vi "LockinRead.vi"() -> ()   [LabVIEW 2019]
uses:
  SineGlobals.vi
panel:
  out "SENS?":dbl
  out "Freq":dbl
  out "Time Const":dbl
  in  "Query":bool
  out "R [Ohm]":dbl
  in  "Auto Gain":bool
  in  "Auto Phase":bool
  in  "Abort":bool
  in  "Arm":bool
  in  "Peak Amp":dbl=1e-05 format="%#_6e"
  in  "Freq":dbl=71.34 format="%#_6e"
  in  "Numeric":i32=300
  out "Waveform Chart":dbl(graph)
  in  "Lockin Name":refnum<visa-resource-name>="GPIB1::8::INSTR"
  in  "Measure":bool
  out "read buffer":string
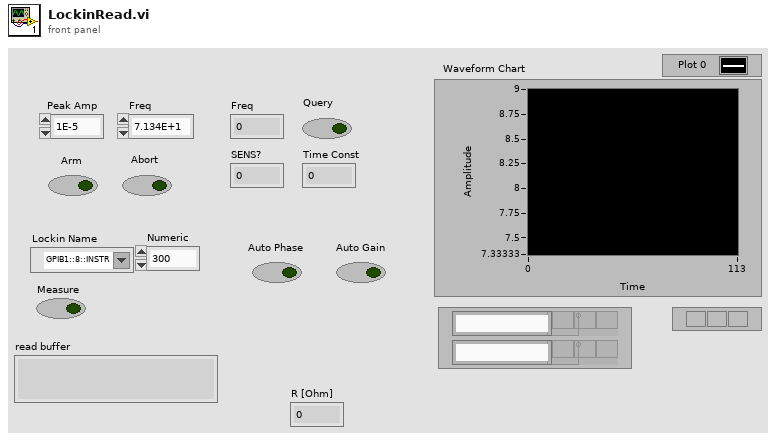
[diagram p1: front panel]
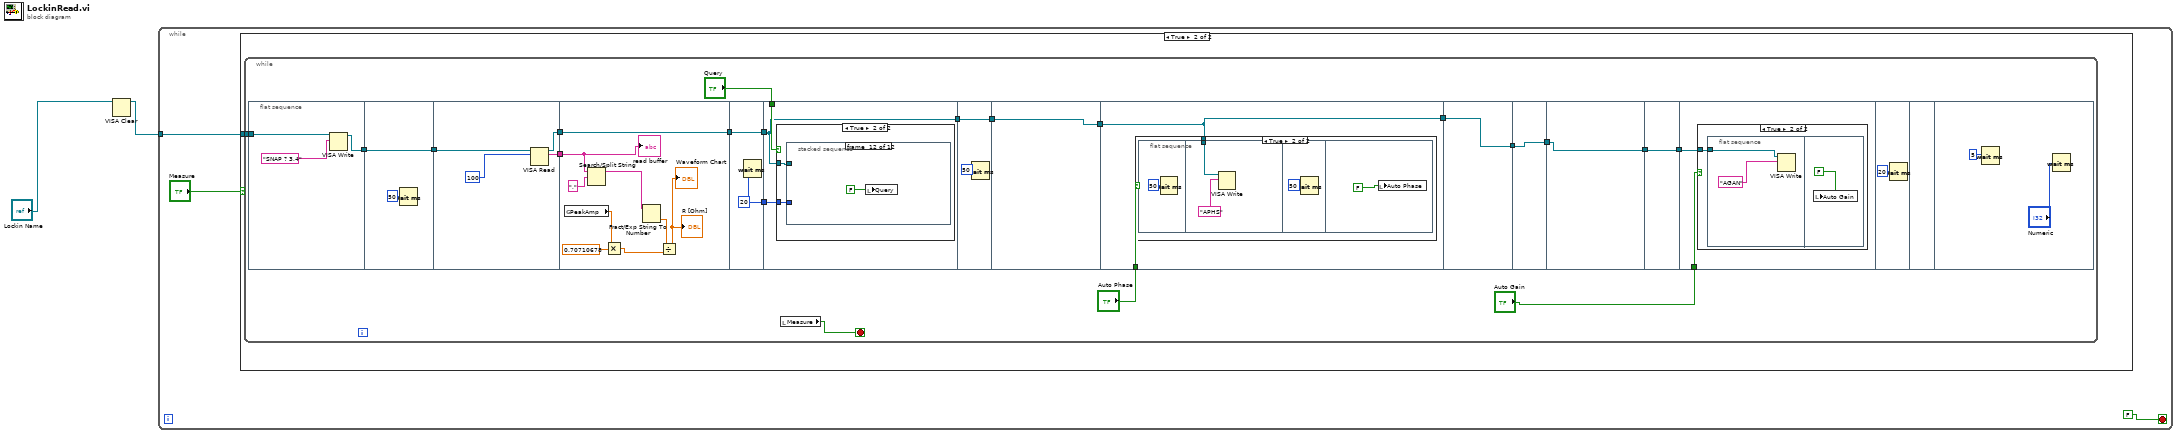
[diagram p0: block diagram]
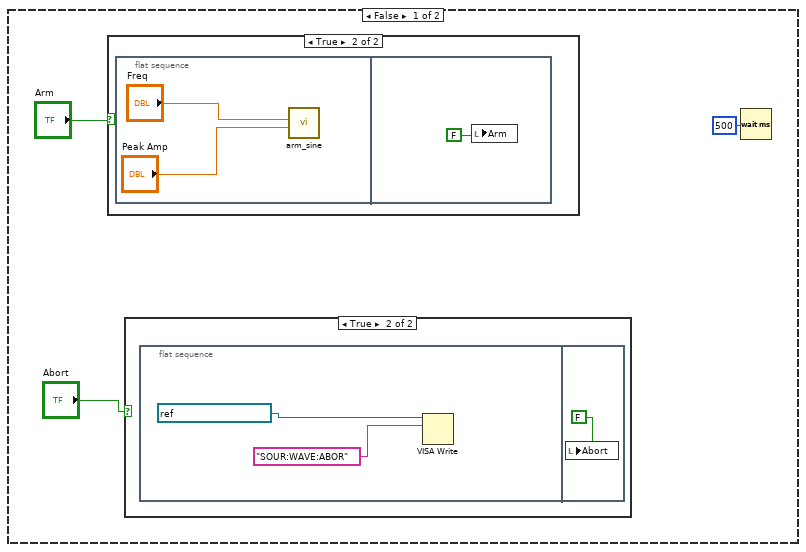
[diagram p2: hidden frame]
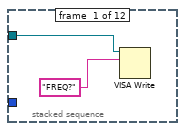
[diagram p6: hidden frame]
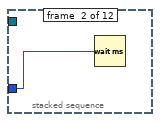
[diagram p7: hidden frame]
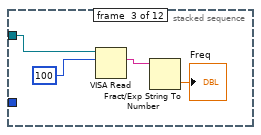
[diagram p8: hidden frame]
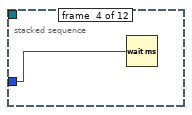
[diagram p9: hidden frame]
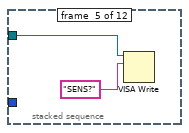
[diagram p10: hidden frame]
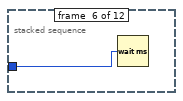
[diagram p11: hidden frame]
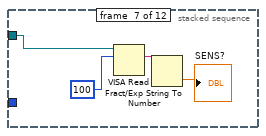
[diagram p12: hidden frame]
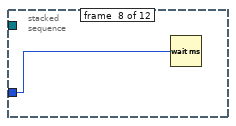
[diagram p13: hidden frame]
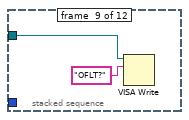
[diagram p14: hidden frame]
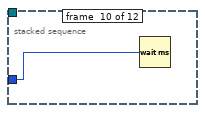
[diagram p15: hidden frame]
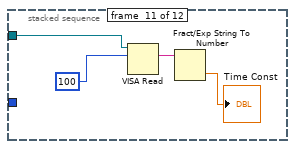
[diagram p16: hidden frame]
diagram:
  n1 = VISA Clear(VISA resource name="Lockin Name") -> (VISA resource name out=w2:refnum<visa-resource-name>)  [unwired: 1 in, 1 out]
  n2 = while {
    tunnel: w2 -> [w3]
    stop <- FALSE stop-if-true
    n3 = case shown="True" "Measure" {
      tunnel: w3 -> [_ w15]
      frame False {
        n4 = case shown="True" "Arm" {
          frame False {
          }
          frame True {
            n5 = flat-sequence {
              frame #0 {
                n6 = call "arm_sine.vi"("Peak Amp"="Peak Amp", "Freq"="Freq") -> ()  [unwired: 10 in]
              }
              frame #1 {
                n7 = local write "Arm"(FALSE) -> ()
              }
            }
          }
        }
        n8 = case shown="True" "Abort" {
          frame False {
          }
          frame True {
            n9 = flat-sequence {
              frame #0 {
                n10 = VISA Write(VISA resource name=refnum<visa-resource-name> "GPIB1::20::INSTR" ("Keithley"), write buffer="SOUR:WAVE:ABOR") -> ()  [unwired: 1 in, 3 out]
              }
              frame #1 {
                n11 = local write "Abort"(FALSE) -> ()
              }
            }
          }
        }
        n12 = Wait (ms)(milliseconds to wait=500) -> ()  [unwired: 1 out]
      }
      frame True {
        n13 = while {
          tunnel: w15 -> [w35]
          stop <- w31 stop-if-true
          n14 = flat-sequence {
            tunnel: w35 -> [w37]
            tunnel: [w36] -> w33
            tunnel: [w40] -> w34
            tunnel: w33 -> [w40]
            tunnel: w34 -> [w44]
            tunnel: [w42] -> w32
            tunnel: [w41] -> w30
            tunnel: w32 -> [w53]
            tunnel: w30 -> [w45]
            tunnel: [w45] -> w29
            tunnel: w29 -> [w55]
            tunnel: [w55] -> w28
            tunnel: [w54] -> w19
            tunnel: w28 -> [w56]
            tunnel: "Query" -> [w58]
            tunnel: w19 -> [w57]
            tunnel: [w56] -> w17
            tunnel: [w85] -> w18
            tunnel: w17 -> [w85]
            tunnel: [w87] -> w27
            tunnel: w18 -> [w87]
            tunnel: w27 -> [w88]
            tunnel: "Auto Phase" -> [w89]
            tunnel: [w88] -> w25
            tunnel: w25 -> [w96]
            tunnel: [w96] -> w16
            tunnel: [w97] -> w24
            tunnel: w16 -> [w97]
            tunnel: w24 -> [w98]
            tunnel: [w98] -> w23
            tunnel: w23 -> [w99]
            tunnel: [w99] -> w22
            tunnel: "Auto Gain" -> [w101]
            tunnel: w22 -> [w100]
            frame #0 {
              n15 = VISA Write(VISA resource name=w37, write buffer="SNAP ? 3,4") -> (VISA resource name out=w36:refnum<visa-resource-name>)  [unwired: 1 in, 2 out]
            }
            frame #1 {
              n16 = Wait (ms)(milliseconds to wait=50) -> ()  [unwired: 1 out]
            }
            frame #2 {
              n17 = VISA Read(VISA resource name=w44, byte count=100) -> (VISA resource name out=w41:refnum<visa-resource-name>, read buffer=w42:string)  [unwired: 1 in, 2 out]
            }
            frame #3 {
              n18 = global read "SineGlobals.vi" "PeakAmp"() -> (w49:dbl)
              n19 = Search/Split String(string=w53, search string/char (-)=",") -> (substring before match=w51:string)  [unwired: 1 in, 2 out]
              n20 = Multiply(x=w49, y=0.70710678) -> (x*y=w46:dbl)
              n21 = Fract/Exp String To Number(string=w51) -> (number=w48:dbl)  [unwired: 3 in, 1 out]
              n22 = Divide(x=w48, y=w46) -> (x/y=→"Waveform Chart" →"R [Ohm]":dbl)
              "read buffer" <- w53
            }
            frame #4 {
              w54 = 20
              n23 = Wait (ms)(milliseconds to wait=w54) -> ()  [unwired: 1 out]
            }
            frame #5 {
              n24 = case shown="True" w58 {
                tunnel: w56 -> [_ w60]
                tunnel: w57 -> [_ w59]
                frame False {
                }
                frame True {
                  n25 = stacked-sequence {
                    tunnel: w60 -> [w61 _ w67 _ w69 _ w75 _ w77 _ w82 _]
                    tunnel: w59 -> [_ w63 _ w68 _ w71 _ w76 _ w79 _ _]
                    frame #0 {
                      n26 = VISA Write(VISA resource name=w61, write buffer="FREQ?") -> ()  [unwired: 1 in, 3 out]
                    }
                    frame #1 {
                      n27 = Wait (ms)(milliseconds to wait=w63) -> ()  [unwired: 1 out]
                    }
                    frame #2 {
                      n28 = VISA Read(VISA resource name=w67, byte count=100) -> (read buffer=w65:string)  [unwired: 1 in, 3 out]
                      n29 = Fract/Exp String To Number(string=w65) -> (number=→"Freq":dbl)  [unwired: 3 in, 1 out]
                    }
                    frame #3 {
                      n30 = Wait (ms)(milliseconds to wait=w68) -> ()  [unwired: 1 out]
                    }
                    frame #4 {
                      n31 = VISA Write(VISA resource name=w69, write buffer="SENS?") -> ()  [unwired: 1 in, 3 out]
                    }
                    frame #5 {
                      n32 = Wait (ms)(milliseconds to wait=w71) -> ()  [unwired: 1 out]
                    }
                    frame #6 {
                      n33 = VISA Read(VISA resource name=w75, byte count=100) -> (read buffer=w73:string)  [unwired: 1 in, 3 out]
                      n34 = Fract/Exp String To Number(string=w73) -> (number=→"SENS?":dbl)  [unwired: 3 in, 1 out]
                    }
                    frame #7 {
                      n35 = Wait (ms)(milliseconds to wait=w76) -> ()  [unwired: 1 out]
                    }
                    frame #8 {
                      n36 = VISA Write(VISA resource name=w77, write buffer="OFLT?") -> ()  [unwired: 1 in, 3 out]
                    }
                    frame #9 {
                      n37 = Wait (ms)(milliseconds to wait=w79) -> ()  [unwired: 1 out]
                    }
                    frame #10 {
                      n38 = VISA Read(VISA resource name=w82, byte count=100) -> (read buffer=w81:string)  [unwired: 1 in, 3 out]
                      n39 = Fract/Exp String To Number(string=w81) -> (number=→"Time Const":dbl)  [unwired: 3 in, 1 out]
                    }
                    frame #11 {
                      n40 = local write "Query"(FALSE) -> ()
                    }
                  }
                }
              }
            }
            frame #6 {
              n41 = Wait (ms)(milliseconds to wait=50) -> ()  [unwired: 1 out]
            }
            frame #7 {
            }
            frame #8 {
              n42 = case shown="True" w89 {
                tunnel: w88 -> [_ w90]
                frame False {
                }
                frame True {
                  n43 = flat-sequence {
                    tunnel: w90 -> [w93]
                    frame #0 {
                      n44 = Wait (ms)(milliseconds to wait=50) -> ()  [unwired: 1 out]
                    }
                    frame #1 {
                      n45 = VISA Write(VISA resource name=w93, write buffer="APHS") -> ()  [unwired: 1 in, 3 out]
                    }
                    frame #2 {
                      n46 = Wait (ms)(milliseconds to wait=50) -> ()  [unwired: 1 out]
                    }
                    frame #3 {
                      n47 = local write "Auto Phase"(FALSE) -> ()
                    }
                  }
                }
              }
            }
            frame #9 {
            }
            frame #10 {
            }
            frame #11 {
            }
            frame #12 {
            }
            frame #13 {
              n48 = case shown="True" w101 {
                tunnel: w100 -> [_ w102]
                frame False {
                }
                frame True {
                  n49 = flat-sequence {
                    tunnel: w102 -> [w104]
                    frame #0 {
                      n50 = VISA Write(VISA resource name=w104, write buffer="AGAN") -> ()  [unwired: 1 in, 3 out]
                    }
                    frame #1 {
                      n51 = local write "Auto Gain"(FALSE) -> ()
                    }
                  }
                }
              }
            }
            frame #14 {
              n52 = Wait (ms)(milliseconds to wait=20) -> ()  [unwired: 1 out]
            }
            frame #15 {
            }
            frame #16 {
              n53 = Wait (ms)(milliseconds to wait=5) -> ()  [unwired: 1 out]
              n54 = Wait (ms)(milliseconds to wait="Numeric") -> ()  [unwired: 1 out]
            }
          }
          n55 = local read "Measure"() -> (w31:bool)
        }
      }
    }
  }
